vi "Bubble Sort Person Array Using Channel Closure.vi"(4 "outputs":T2, 11 "Unsorted":T3[](array[typedef]) {"Birth Date" format="%<%Y/%b/%d>T"}) -> (3 "Sorted":T3[](array[typedef]) {"Birth Date" format="%<%Y/%b/%d>T"}, 6 "inputs":T1)   [LabVIEW 2023]
doc: "This VI implements a basic Bubble Sort for the array data, using the provided VI reference as the comparison function for two elements."
uses:
  Person Information.ctl
  <extravilib>/ChannelInstances/One Element Stream-bool/)Channel.ctl
  <extravilib>/ChannelInstances/One Element Stream-t'Person Compare Closure Inputs.ctl'/)Channel.ctl
  Person Compare Closure Inputs.ctl
  <extravilib>/ChannelInstances/One Element Stream-t'Person Compare Closure Inputs.ctl'/Write With Abort.vi
  <extravilib>/ChannelInstances/One Element Stream-bool/Read With Abort.vi
  <extravilib>/ChannelInstances/One Element Stream-t'Person Compare Closure Inputs.ctl'/Endpoint.vi
  <extravilib>/ChannelInstances/One Element Stream-bool/EndpointRead.vi
  <extravilib>/ChannelInstances/One Element Stream-bool.lvlib
  <extravilib>/ChannelInstances/One Element Stream-t'Person Compare Closure Inputs.ctl'.lvlib
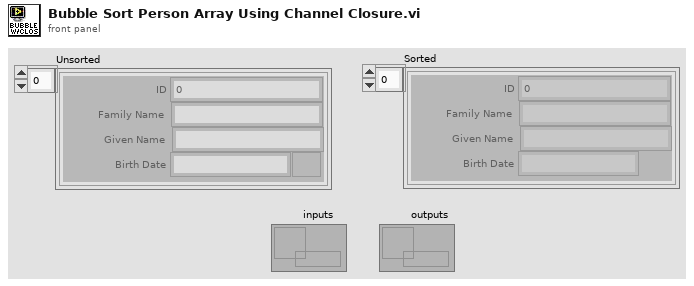
[diagram p1: front panel]
types:
  T1 = typedef "One Element Stream-t'Person Compare Closure Inputs.ctl'.lvlib/)Channel.ctl" = refnum<queue>
  T2 = typedef "One Element Stream-bool.lvlib/)Channel.ctl" = refnum<queue>
  T3 = typedef "Person Information.ctl" = cluster{"ID":u32, "Family Name":string, "Given Name":string, "Birth Date":timestamp}
  T4 = typedef "Person Compare Closure Inputs.ctl" = cluster{"Person A":T3, "Person B":T3}
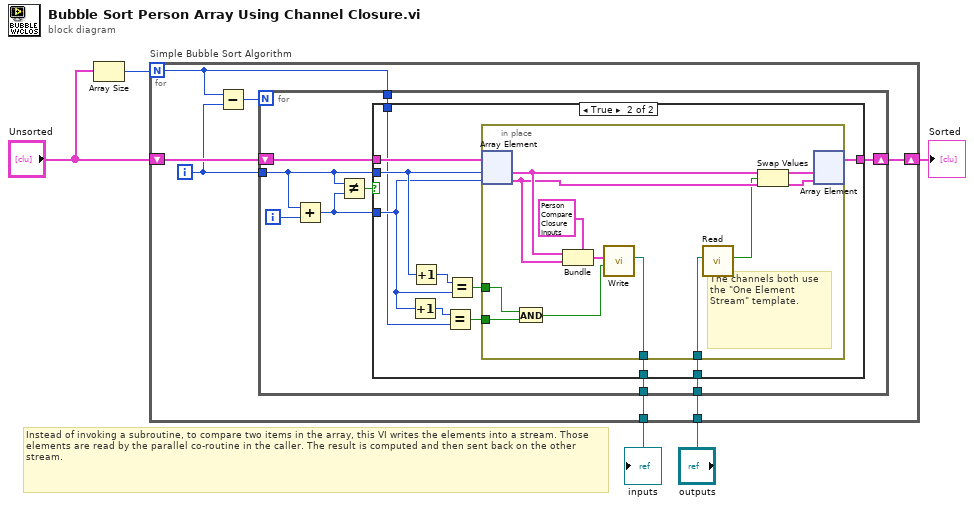
[diagram p0: block diagram]
diagram:
  # "Instead of invoking a subroutine, to compare two items in the array, this VI writes the elements into a stream. Those elements are read by the parallel co-routine in the caller. The result is computed and then sent back on the other stream."
  n1 = Array Size(array="Unsorted") -> (size(s)=w1:i32)
  n2 = for "Simple Bubble Sort Algorithm" {
    N: w1 -> [w6]
    shift-right: [w11] -> w5
    shift-left: "Unsorted" -> [w12]
    tunnel: "outputs" -> [w10]
    tunnel: [w9] -> w2
    i -> [w8]
    n3 = Subtract(x=w6, y=w8) -> (x-y=w7:i32)
    n4 = for {
      N: w7 -> [_]
      shift-right: [w20] -> w11
      shift-left: w12 -> [w21]
      tunnel: w8 -> [w17]
      tunnel: w10 -> [w16]
      tunnel: [w15] -> w9
      tunnel: w6 -> [w13]
      i -> [w14]
      n5 = Add(x=w17, y=w14) -> (x+y=w18:i32)
      n6 = Not Equal?(x=w17, y=w18) -> (x != y?=w19:bool)
      n7 = case shown="True" w19 {
        tunnel: w21 -> [w22 w33]
        tunnel: [w22 w32] -> w20
        tunnel: w17 -> [_ w29]
        tunnel: w18 -> [_ w27]
        tunnel: w16 -> [_ w31]
        tunnel: [_ w30] -> w15
        tunnel: w13 -> [_ w25]
        frame False {
        }
        frame True {
          n8 = Increment(x=w27) -> (x+1=w26:i32)
          n9 = Increment(x=w29) -> (x+1=w28:i32)
          n10 = Equal?(x=w26, y=w25) -> (x = y?=w23:bool)
          n11 = Equal?(x=w28, y=w27) -> (x = y?=w24:bool)
          n12 = in-place {
            in-place-border: w31 -> [w39]
            in-place-border: [w37] -> w30
            in-place-border: w24 -> [w36]
            in-place-border: w23 -> [w35]
            # "The channels both use the \"One Element Stream\" template."
            n13 = in-place-array #1(w33, w29, w27) -> (w43:T3, w42:T3)
            n14 = And(x=w36, y=w35) -> (x .and. y?=w34:bool)
            n15 = Bundle(cluster=T4 {"Person A"={"ID"=0, "Family Name"="", "Given Name"="", "Birth Date"=timestamp(0 s since 1904-01-01)}, "Person B"={"ID"=0, "Family Name"="", "Given Name"="", "Birth Date"=timestamp(0 s since 1904-01-01)}} ("inputs"), "Person A"=w43, "Person B"=w42) -> (w40:T4)
            n16 = call <extravilib>:"Write.vi"("last element? (F)"=w34, "element"=w40) -> ("channel"=w37:T1)  [unwired: 8 in, 1 out]
            n17 = call <extravilib>:"Read.vi"("channel"=w39) -> ("element"=w38:bool)  [unwired: 7 in, 3 out]
            n18 = Swap Values(12:w43, 13:w38, 14:w42) -> (1:w45:T3, 3:w44:T3)
            n19 = in-place-array #1(w45, w44) -> (w32:T3[])  [unwired: 2 out]
          }
        }
      }
    }
  }
  "Sorted" <- w5
  "inputs" <- w2
